vi "EventLogger.Close.vi"(8 "error in":errorcluster) -> (0 "error out":errorcluster)   [LabVIEW 2019, in "Tools.lvlib"]
uses:
  Tools.lvlib
  EventLogger.Manager.Action.ctl
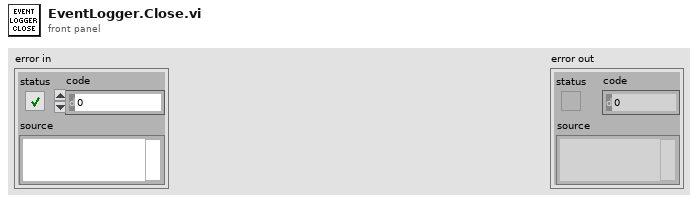
[diagram p1: front panel]
types:
  T1 = typedef "Tools.lvlib/EventLogger.Manager.Action.ctl" = enum16{"init", "get", "close"}
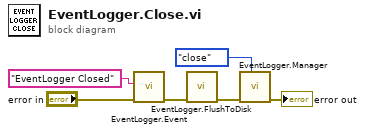
[diagram p0: block diagram]
diagram:
  n1 = call "EventLogger.Event.vi"("error in"="error in", "Event Name"="EventLogger Closed") -> ("error out"=w3:errorcluster)  [unwired: 9 in]
  n2 = call "EventLogger.FlushToDisk.vi"("error in"=w3) -> ("error out"=w1:errorcluster)  [unwired: 10 in]
  n3 = call "EventLogger.Manager.vi"("action"=EventLogger.Manager.Action."close", "error in"=w1) -> ("error out"=→"error out":errorcluster)  [unwired: 8 in, 1 out]
